vi "sub_gauss-likelihood.vi"(10 "sigma":dbl, 11 "x":dbl) -> (3 "p":dbl)   [LabVIEW 2019]
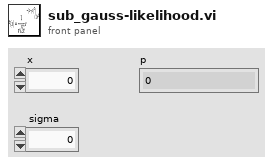
[diagram p1: front panel]
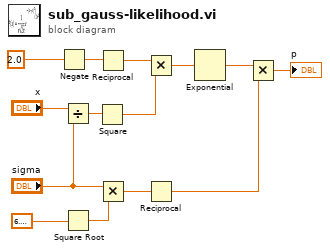
[diagram p0: block diagram]
diagram:
  n1 = Negate(x=2.0) -> (-x=w10:dbl)
  n2 = Divide(x="x", y="sigma") -> (x/y=w7:dbl)
  n3 = Square Root(x=6.283185307179586) -> (sqrt(x)=w13:dbl)
  n4 = Square(x=w7) -> (x^2=w6:dbl)
  n5 = Reciprocal(x=w10) -> (1/x=w5:dbl)
  n6 = Multiply(x="sigma", y=w13) -> (x*y=w12:dbl)
  n7 = Multiply(x=w5, y=w6) -> (x*y=w4:dbl)
  n8 = Reciprocal(x=w12) -> (1/x=w2:dbl)
  n9 = Exponential(1:w4) -> (0:w3:dbl)
  n10 = Multiply(x=w3, y=w2) -> (x*y=→"p":dbl)
